vi "Circle Info.vi"(8 "Circles Data (Circle Detection 1) 2":T3(array[cluster]), 11 "Chosen Particle Info 2":T2) -> (0 "Ordered Pairs":T1, 3 "Number of Pairs":i32)   [LabVIEW 2012]
uses:
  <vilib>/Analysis/Matrix/Datatypes/RealMatrix.ctl
  <vilib>/Analysis/Matrix/NI_Matrix.lvlib
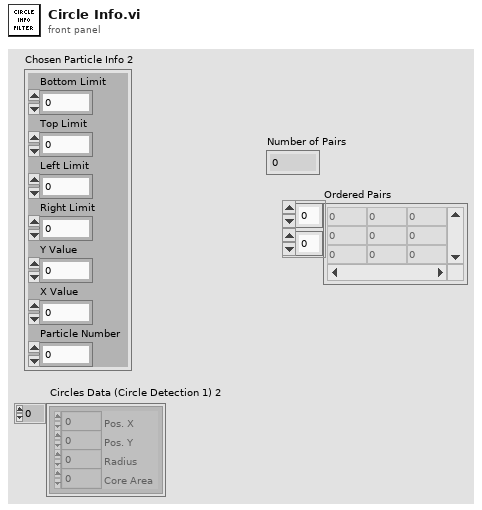
[diagram p1: front panel]
types:
  T1 = typedef "NI_Matrix.lvlib/RealMatrix.ctl" = dbl[][]
  T2 = cluster{"Bottom Limit":i32, "Top Limit":i32, "Left Limit":i32, "Right Limit":i32, "Y Value":i32, "X Value":i32, "Particle Number":i32}
  T3 = cluster{"Pos. X":i32, "Pos. Y":i32, "Radius":i32, "Core Area":i32}[]
  T4 = cluster{"Circles Data (Circle Detection 1) 2[0]":cluster{"Pos. X":i32, "Pos. Y":i32, "Radius":i32, "Core Area":i32}, "Circles Data (Circle Detection 1) 2[1]":cluster{"Pos. X":i32, "Pos. Y":i32, "Radius":i32, "Core Area":i32}, "Circles Data (Circle Detection 1) 2[2]":cluster{"Pos. X":i32, "Pos. Y":i32, "Radius":i32, "Core Area":i32}, "Circles Data (Circle Detection 1) 2[3]":cluster{"Pos. X":i32, "Pos. Y":i32, "Radius":i32, "Core Area":i32}, "Circles Data (Circle Detection 1) 2[4]":cluster{"Pos. X":i32, "Pos. Y":i32, "Radius":i32, "Core Area":i32}, "Circles Data (Circle Detection 1) 2[5]":cluster{"Pos. X":i32, "Pos. Y":i32, "Radius":i32, "Core Area":i32}, "Circles Data (Circle Detection 1) 2[6]":cluster{"Pos. X":i32, "Pos. Y":i32, "Radius":i32, "Core Area":i32}, "Circles Data (Circle Detection 1) 2[7]":cluster{"Pos. X":i32, "Pos. Y":i32, "Radius":i32, "Core Area":i32}, "Circles Data (Circle Detection 1) 2[8]":cluster{"Pos. X":i32, "Pos. Y":i32, "Radius":i32, "Core Area":i32}}
  T5 = cluster{"Pos. X":i32, "Pos. Y":i32, "Radius":i32, "Core Area":i32}
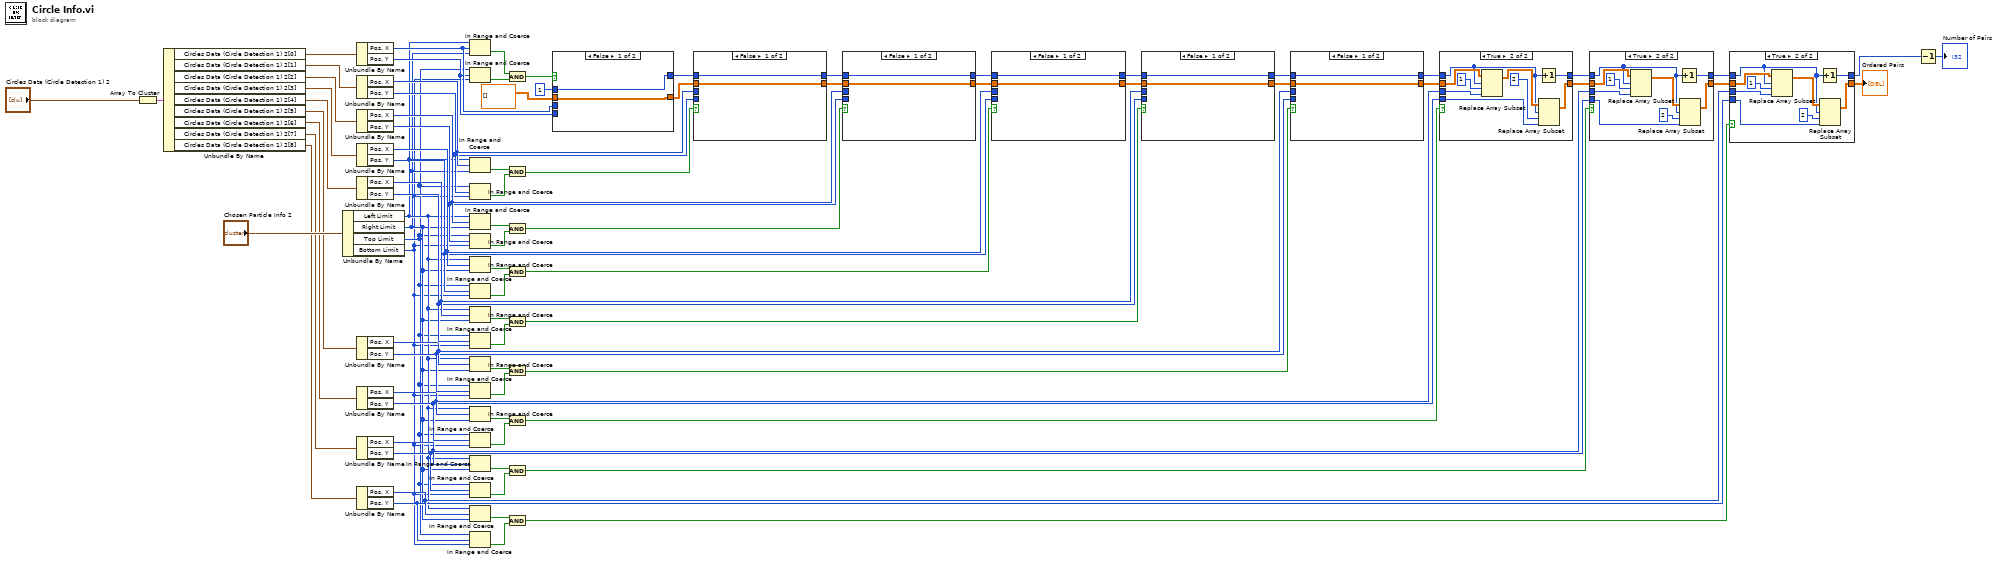
[diagram p0: block diagram]
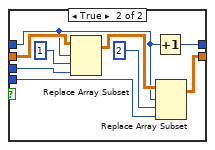
[diagram p5: hidden frame]
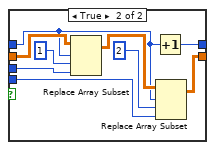
[diagram p6: hidden frame]
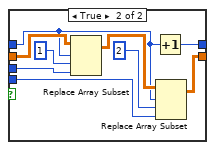
[diagram p7: hidden frame]
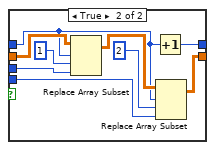
[diagram p8: hidden frame]
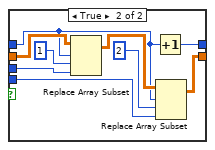
[diagram p9: hidden frame]
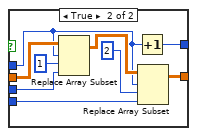
[diagram p10: hidden frame]
diagram:
  n1 = Array To Cluster(array="Circles Data (Circle Detection 1) 2") -> (cluster=w80:T4)
  n2 = Unbundle By Name(w80) -> ("Circles Data (Circle Detection 1) 2[0]"=w79:T5, "Circles Data (Circle Detection 1) 2[1]"=w24:T5, "Circles Data (Circle Detection 1) 2[2]"=w23:T5, "Circles Data (Circle Detection 1) 2[3]"=w22:T5, "Circles Data (Circle Detection 1) 2[4]"=w20:T5, "Circles Data (Circle Detection 1) 2[5]"=w19:T5, "Circles Data (Circle Detection 1) 2[6]"=w18:T5, "Circles Data (Circle Detection 1) 2[7]"=w17:T5, "Circles Data (Circle Detection 1) 2[8]"=w9:T5)
  n3 = Unbundle By Name("Chosen Particle Info 2") -> ("Left Limit"=w8:i32, "Right Limit"=w7:i32, "Top Limit"=w6:i32, "Bottom Limit"=w5:i32)
  n4 = Unbundle By Name(w79) -> ("Pos. X"=w75:i32, "Pos. Y"=w74:i32)
  n5 = Unbundle By Name(w24) -> ("Pos. X"=w69:i32, "Pos. Y"=w68:i32)
  n6 = Unbundle By Name(w23) -> ("Pos. X"=w64:i32, "Pos. Y"=w63:i32)
  n7 = Unbundle By Name(w22) -> ("Pos. X"=w59:i32, "Pos. Y"=w58:i32)
  n8 = Unbundle By Name(w20) -> ("Pos. X"=w54:i32, "Pos. Y"=w53:i32)
  n9 = Unbundle By Name(w19) -> ("Pos. X"=w49:i32, "Pos. Y"=w48:i32)
  n10 = Unbundle By Name(w18) -> ("Pos. X"=w44:i32, "Pos. Y"=w43:i32)
  n11 = Unbundle By Name(w17) -> ("Pos. X"=w39:i32, "Pos. Y"=w38:i32)
  n12 = Unbundle By Name(w9) -> ("Pos. X"=w13:i32, "Pos. Y"=w12:i32)
  n13 = In Range and Coerce(upper limit=w8, x=w75, lower limit=w7) -> (In Range?=w78:bool)  [unwired: 1 out]
  n14 = In Range and Coerce(upper limit=w6, x=w74, lower limit=w5) -> (In Range?=w77:bool)  [unwired: 1 out]
  n15 = In Range and Coerce(upper limit=w8, x=w69, lower limit=w7) -> (In Range?=w72:bool)  [unwired: 1 out]
  n16 = In Range and Coerce(upper limit=w6, x=w68, lower limit=w5) -> (In Range?=w71:bool)  [unwired: 1 out]
  n17 = In Range and Coerce(upper limit=w8, x=w64, lower limit=w7) -> (In Range?=w67:bool)  [unwired: 1 out]
  n18 = In Range and Coerce(upper limit=w6, x=w63, lower limit=w5) -> (In Range?=w66:bool)  [unwired: 1 out]
  n19 = In Range and Coerce(upper limit=w8, x=w59, lower limit=w7) -> (In Range?=w62:bool)  [unwired: 1 out]
  n20 = In Range and Coerce(upper limit=w6, x=w58, lower limit=w5) -> (In Range?=w61:bool)  [unwired: 1 out]
  n21 = In Range and Coerce(upper limit=w8, x=w54, lower limit=w7) -> (In Range?=w57:bool)  [unwired: 1 out]
  n22 = In Range and Coerce(upper limit=w6, x=w53, lower limit=w5) -> (In Range?=w56:bool)  [unwired: 1 out]
  n23 = In Range and Coerce(upper limit=w8, x=w49, lower limit=w7) -> (In Range?=w52:bool)  [unwired: 1 out]
  n24 = In Range and Coerce(upper limit=w6, x=w48, lower limit=w5) -> (In Range?=w51:bool)  [unwired: 1 out]
  n25 = In Range and Coerce(upper limit=w8, x=w44, lower limit=w7) -> (In Range?=w47:bool)  [unwired: 1 out]
  n26 = In Range and Coerce(upper limit=w6, x=w43, lower limit=w5) -> (In Range?=w46:bool)  [unwired: 1 out]
  n27 = In Range and Coerce(upper limit=w8, x=w39, lower limit=w7) -> (In Range?=w42:bool)  [unwired: 1 out]
  n28 = In Range and Coerce(upper limit=w6, x=w38, lower limit=w5) -> (In Range?=w41:bool)  [unwired: 1 out]
  n29 = In Range and Coerce(upper limit=w8, x=w13, lower limit=w7) -> (In Range?=w16:bool)  [unwired: 1 out]
  n30 = In Range and Coerce(upper limit=w6, x=w12, lower limit=w5) -> (In Range?=w15:bool)  [unwired: 1 out]
  n31 = And(x=w78, y=w77) -> (x .and. y?=w76:bool)
  n32 = And(x=w72, y=w71) -> (x .and. y?=w70:bool)
  n33 = And(x=w67, y=w66) -> (x .and. y?=w65:bool)
  n34 = And(x=w62, y=w61) -> (x .and. y?=w60:bool)
  n35 = And(x=w57, y=w56) -> (x .and. y?=w55:bool)
  n36 = And(x=w52, y=w51) -> (x .and. y?=w50:bool)
  n37 = And(x=w47, y=w46) -> (x .and. y?=w45:bool)
  n38 = And(x=w42, y=w41) -> (x .and. y?=w40:bool)
  n39 = And(x=w16, y=w15) -> (x .and. y?=w14:bool)
  n40 = case shown="False" w76 {
    tunnel: w75 -> [_ w89]
    tunnel: w74 -> [_ w88]
    tunnel: T1 [] ("matrix") -> [w84 w93]
    tunnel: [w84 w87] -> w37
    tunnel: 1 -> [w83 w86]
    tunnel: [w83 w85] -> w36
    frame False {
    }
    frame True {
      n41 = Replace Array Subset(array=w93, new element=w89, index (row)=w86, index (col)=1) -> (w92:T1)
      n42 = Increment(x=w86) -> (x+1=w85:i32)
      n43 = Replace Array Subset(array=w92, new element=w88, index (row)=w86, index (col)=2) -> (w87:T1)
    }
  }
  n44 = case shown="False" w70 {
    tunnel: w69 -> [_ w100]
    tunnel: w68 -> [_ w99]
    tunnel: w37 -> [w95 w104]
    tunnel: [w95 w98] -> w35
    tunnel: w36 -> [w94 w97]
    tunnel: [w94 w96] -> w34
    frame False {
    }
    frame True {
      n45 = Replace Array Subset(array=w104, new element=w100, index (row)=w97, index (col)=1) -> (w103:T1)
      n46 = Increment(x=w97) -> (x+1=w96:i32)
      n47 = Replace Array Subset(array=w103, new element=w99, index (row)=w97, index (col)=2) -> (w98:T1)
    }
  }
  n48 = case shown="False" w65 {
    tunnel: w64 -> [_ w111]
    tunnel: w63 -> [_ w110]
    tunnel: w35 -> [w106 w115]
    tunnel: [w106 w109] -> w33
    tunnel: w34 -> [w105 w108]
    tunnel: [w105 w107] -> w32
    frame False {
    }
    frame True {
      n49 = Replace Array Subset(array=w115, new element=w111, index (row)=w108, index (col)=1) -> (w114:T1)
      n50 = Increment(x=w108) -> (x+1=w107:i32)
      n51 = Replace Array Subset(array=w114, new element=w110, index (row)=w108, index (col)=2) -> (w109:T1)
    }
  }
  n52 = case shown="False" w60 {
    tunnel: w59 -> [_ w122]
    tunnel: w58 -> [_ w121]
    tunnel: w33 -> [w117 w126]
    tunnel: [w117 w120] -> w21
    tunnel: w32 -> [w116 w119]
    tunnel: [w116 w118] -> w31
    frame False {
    }
    frame True {
      n53 = Replace Array Subset(array=w126, new element=w122, index (row)=w119, index (col)=1) -> (w125:T1)
      n54 = Increment(x=w119) -> (x+1=w118:i32)
      n55 = Replace Array Subset(array=w125, new element=w121, index (row)=w119, index (col)=2) -> (w120:T1)
    }
  }
  n56 = case shown="False" w55 {
    tunnel: w54 -> [_ w133]
    tunnel: w53 -> [_ w132]
    tunnel: w21 -> [w128 w137]
    tunnel: [w128 w131] -> w30
    tunnel: w31 -> [w127 w130]
    tunnel: [w127 w129] -> w29
    frame False {
    }
    frame True {
      n57 = Replace Array Subset(array=w137, new element=w133, index (row)=w130, index (col)=1) -> (w136:T1)
      n58 = Increment(x=w130) -> (x+1=w129:i32)
      n59 = Replace Array Subset(array=w136, new element=w132, index (row)=w130, index (col)=2) -> (w131:T1)
    }
  }
  n60 = case shown="False" w50 {
    tunnel: w49 -> [_ w144]
    tunnel: w48 -> [_ w143]
    tunnel: w30 -> [w139 w148]
    tunnel: [w139 w142] -> w28
    tunnel: w29 -> [w138 w141]
    tunnel: [w138 w140] -> w27
    frame False {
    }
    frame True {
      n61 = Replace Array Subset(array=w148, new element=w144, index (row)=w141, index (col)=1) -> (w147:T1)
      n62 = Increment(x=w141) -> (x+1=w140:i32)
      n63 = Replace Array Subset(array=w147, new element=w143, index (row)=w141, index (col)=2) -> (w142:T1)
    }
  }
  n64 = case shown="True" w45 {
    tunnel: w44 -> [_ w155]
    tunnel: w43 -> [_ w154]
    tunnel: w28 -> [w150 w159]
    tunnel: [w150 w153] -> w26
    tunnel: w27 -> [w149 w152]
    tunnel: [w149 w151] -> w25
    frame False {
    }
    frame True {
      n65 = Replace Array Subset(array=w159, new element=w155, index (row)=w152, index (col)=1) -> (w158:T1)
      n66 = Increment(x=w152) -> (x+1=w151:i32)
      n67 = Replace Array Subset(array=w158, new element=w154, index (row)=w152, index (col)=2) -> (w153:T1)
    }
  }
  n68 = case shown="True" w40 {
    tunnel: w39 -> [_ w166]
    tunnel: w38 -> [_ w165]
    tunnel: w26 -> [w161 w170]
    tunnel: [w161 w164] -> w11
    tunnel: w25 -> [w160 w163]
    tunnel: [w160 w162] -> w10
    frame False {
    }
    frame True {
      n69 = Replace Array Subset(array=w170, new element=w166, index (row)=w163, index (col)=1) -> (w169:T1)
      n70 = Increment(x=w163) -> (x+1=w162:i32)
      n71 = Replace Array Subset(array=w169, new element=w165, index (row)=w163, index (col)=2) -> (w164:T1)
    }
  }
  n72 = case shown="True" w14 {
    tunnel: w13 -> [_ w177]
    tunnel: w12 -> [_ w176]
    tunnel: w11 -> [w172 w181]
    tunnel: [w172 w175] -> w2
    tunnel: w10 -> [w171 w174]
    tunnel: [w171 w173] -> w4
    frame False {
    }
    frame True {
      n73 = Replace Array Subset(array=w181, new element=w177, index (row)=w174, index (col)=1) -> (w180:T1)
      n74 = Increment(x=w174) -> (x+1=w173:i32)
      n75 = Replace Array Subset(array=w180, new element=w176, index (row)=w174, index (col)=2) -> (w175:T1)
    }
  }
  "Ordered Pairs" <- w2
  n76 = Decrement(x=w4) -> (x-1=→"Number of Pairs":i32)
